vi "HFRR ADV v01.vi"() -> ()   [LabVIEW 2023] (continued)
                n759 = case shown="True" w2095 {
                  tunnel: w2094 -> [_ w2177]
                  tunnel: [FALSE ("Boolean 2") TRUE ("Boolean 2")] -> _
                  frame False {
                  }
                  frame True {
                    w2145 = ";" ("Substring")
                    # "Pid out/\nFreq response value"
                    n760 = local read "Set Strk"() -> (w2144:dbl)
                    n761 = local read "Stroke"() -> (w2134:dbl)
                    n762 = local write "act save time"(w2177) -> ()
                    n763 = Subtract(x=w2134, y=w2144) -> (x-y=w2141:dbl)
                    n764 = Multiply(x=w2141, y=0.05) -> (x*y=w2143:dbl)
                    n765 = local read "Humidity"() -> (w2152:dbl)
                    "gRh" <- w2152
                    n766 = local read "Elapsed time"() -> (w2170:dbl)
                    n767 = local read "COF 2"() -> (w2132:dbl)
                    "cof" <- w2132
                    "Coefficient of Friction" <- w2132
                    n768 = local read "AIR TEMP"() -> (w2133:dbl)
                    n769 = local read "FF 2"() -> (→"Frictional Force ( N )":dbl)
                    n770 = Add(x=w2143, y=w2144) -> (x+y=w2135:dbl)
                    "Stroke Ln" <- w2135
                    "Stroke 2" <- w2135
                    "Disp" <- w2135
                    n771 = local read "TEMP"() -> (w2129:dbl)
                    "Temp" <- w2129
                    "Electronic contact resistance ( % )" <- w2129
                    n772 = local read "ecr"() -> (w2130:dbl)
                    "ecr 2" <- w2130
                    n773 = local write "Electronic contact resistance ( % )"(w2130) -> ()
                    n774 = local read "Hz"() -> (w2137:dbl)
                    n775 = local read "PID-out"() -> (w2140:dbl)
                    n776 = Number To Fractional String(number=w2135, width (-)=i16 9 ("precision (6)"), precision (6)=i16 6) -> (F-format string=w2163:string)  [unwired: 1 in]
                    n777 = Number To Fractional String(number=w2133, width (-)=i16 9 ("precision (6)"), precision (6)=i16 3) -> (F-format string=w2162:string)  [unwired: 1 in]
                    n778 = Number To Fractional String(number=w2170, width (-)=i16 14 ("precision (6)"), precision (6)=i16 3) -> (F-format string=w2172:string)  [unwired: 1 in]
                    n779 = Number To Fractional String(number=w2132, width (-)=i16 9 ("precision (6)"), precision (6)=i16 6) -> (F-format string=w2171:string)  [unwired: 1 in]
                    n780 = Number To Fractional String(number=w2129, width (-)=i16 9 ("precision (6)"), precision (6)=i16 3) -> (F-format string=w2159:string)  [unwired: 1 in]
                    n781 = Number To Fractional String(number=w2152, width (-)=i16 9 ("precision (6)"), precision (6)=i16 3) -> (F-format string=w2156:string)  [unwired: 1 in]
                    n782 = Number To Fractional String(number=w2130, width (-)=i16 9 ("precision (6)"), precision (6)=i16 3) -> (F-format string=w2151:string)  [unwired: 1 in]
                    n783 = Number To Fractional String(number=w2140, width (-)=i16 9 ("precision (6)"), precision (6)=i16 3) -> (F-format string=w2146:string)  [unwired: 1 in]
                    n784 = Number To Fractional String(number=w2137, width (-)=i16 9 ("precision (6)"), precision (6)=i16 3) -> (F-format string=w2136:string)  [unwired: 1 in]
                    n785 = Concatenate Strings(w2172, w2145, w2171, w2145, w2163, w2145, w2162, w2145, w2159, w2145, w2156, w2145, w2151, w2145, w2146, w2145, w2136, "\r") -> (w2169:string)
                    n786 = local read "FILE"() -> (w2178:string)
                    n787 = Concatenate Strings("C:\\LAB-IQ-NXT\\Data\\" ("string"), w2178, ".dgf" ("Substring")) -> (w2180:string)
                    n788 = String To Path(string=w2180) -> (path=w2179:path)
                    n789 = call <vilib>:"Write Characters To File.vi"("append to file? (new file:F)"=TRUE, "character string"=w2169, "file path (dialog if empty)"=w2179) -> ()  [unwired: 2 in, 1 out]
                    "refresh flag" <- TRUE ("refresh flag")
                  }
                }
                n790 = local read "COUNT"() -> (w2087:i32)
                n791 = Multiply(x=w2101, y=w2087) -> (x*y=w2093:dbl)
                n792 = Add(x=w2096, y=w2093) -> (x+y=w2080:dbl)
                "Elapsed time 3" <- w2080
                n793 = local read "Test \nStatus"() -> (w2081:bool)
                n794 = local read "clk"() -> (w2088:dbl)
                n795 = Equal?(x=w2088, y=10.0) -> (x = y?=w2090:bool)
                n796 = Divide(x=w2080, y=60.0) -> (x/y=w2091:dbl)
                n797 = case shown="True" w2081 {
                  tunnel: w2091 -> [_ w2113]
                  tunnel: w2096 -> [_ w2121]
                  tunnel: [0.0 w2117] -> _
                  tunnel: w2090 -> [_ w2116]
                  tunnel: [0.0 w2115] -> _
                  tunnel: w2080 -> [_ w2115]
                  tunnel: w2094 -> [w2109 _]
                  frame False {
                    n798 = local write "acq timer"(w2109) -> ()
                  }
                  frame True {
                    n799 = local read "Set Hz"() -> (w2118:dbl)
                    n800 = local write "Elapsed time"(w2113) -> ()
                    n801 = local read "test time"() -> (w2114:dbl)
                    n802 = Multiply(x=w2121, y=w2118) -> (x*y=w2120:dbl)
                    n803 = case shown="False" w2116 {
                      tunnel: w2120 -> [w2122 _]
                      tunnel: [w2122 1.0] -> w2117
                      frame False {
                        n804 = local write "Cycles elapsed"(w2122) -> ()
                      }
                      frame True {
                      }
                    }
                    n805 = Subtract(x=w2114, y=w2113) -> (x-y=w2112:dbl)
                    "time" <- w2112
                    n806 = Greater?(x=w2113, y=w2114) -> (0:w2119:bool)
                    n807 = case shown="True" w2119 {
                      frame False {
                      }
                      frame True {
                        n808 = local read "Humidity"() -> (→"Rh After":dbl)
                        n809 = property on="STOP 2" class="Bool (strict)"("Disabled"=u8 0) -> ()  [unwired: 2 in, 2 out]
                        n810 = local write "RUN"(FALSE ("OK Button 2")) -> ()
                        n811 = local write "STOP 3"(TRUE ("STOP")) -> ()
                      }
                    }
                    n812 = local write "Time Remaining"(w2112) -> ()
                  }
                }
              }
              frame #2 {
                n813 = case shown="True" "Heater Button" {
                  tunnel: [0.0 ("output") w2204] -> w2183
                  frame False {
                    w2185 = TRUE ("tmpchk")
                    n814 = local write "tmpchk"(w2185) -> ()
                    n815 = local write "Reset 4"(w2185) -> ()
                    n816 = local read "TEMP"() -> (w2186:dbl)
                    n817 = local write "Temp ini"(w2186) -> ()
                    n818 = local write "reinit"(TRUE ("reinit")) -> ()
                  }
                  frame True {
                    # "Logic to turn off\nthe heater when \ntemp is not rising.\nTime - 60 sec\nDelta t- 5°c"
                    n819 = local read "Set Temp"() -> (w2201:dbl)
                    n820 = local read "Temp ini"() -> (w2192:dbl)
                    n821 = local read "TEMP"() -> (w2195:dbl)
                    n822 = Add(x=w2201, y=0.5) -> (x+y=w2199:dbl)
                    n823 = Less?(x=w2192, y=53.0) -> (x < y?=w2190:bool)
                    n824 = Greater Or Equal?(x=w2195, y=w2199) -> ()  [unwired: 1 out]
                    n825 = And(x="tmpchk", y=w2190) -> (x .and. y?=w2193:bool)
                    n826 = case shown="True" w2193 {
                      frame False {
                      }
                      frame True {
                        n827 = call "Elapsed Time8"("Time Target (s)"=300.0, "Reset"="Reset 4") -> ("Time has Elapsed"=w2209:bool)  [unwired: 10 in, 7 out]
                        n828 = flat-sequence {
                          tunnel: w2209 -> [_]
                          frame #0 {
                            n829 = local write "Reset 4"(FALSE ("Reset 4")) -> ()
                          }
                        }
                        n830 = case shown="True" w2209 {
                          frame False {
                          }
                          frame True {
                            n831 = local read "Temp ini"() -> (w2216:dbl)
                            n832 = local read "TEMP"() -> (w2217:dbl)
                            n833 = Add(x=w2216, y=5.0) -> (x+y=w2214:dbl)
                            n834 = Greater?(x=w2217, y=w2214) -> (0:w2215:bool)
                            n835 = case shown="False" w2215 {
                              frame False {
                                n836 = local write "Heater Button"(FALSE ("Heater Button")) -> ()
                              }
                              frame True {
                                n837 = local write "tmpchk"(FALSE ("tmpchk")) -> ()
                              }
                            }
                          }
                        }
                      }
                    }
                    n838 = call-poly <vilib>:"PID.vi"("reinitialize? (F)"="reinit", "output range"="output range", "dt (s)"=-1.0, "PID gains"="Temp PID gains", "process variable"=w2195, "setpoint"=w2201) -> ("output"=w2198:dbl)  [unwired: 4 in, 1 out]
                    n839 = Select(t=0.0, s=FALSE, f=w2198) -> (s? t:f=w2197:dbl)
                    "PID output" <- w2197
                    n840 = Subtract(x=w2201, y=w2195) -> (x-y=w2203:dbl)
                    n841 = flat-sequence {
                      tunnel: w2197 -> [w2220]
                      tunnel: [w2220] -> w2204
                      frame #0 {
                        n842 = local write "reinit"(FALSE ("reinit")) -> ()
                      }
                    }
                    n843 = Bundle(w2203, "output"=w2197, "TEMP"=w2195) -> (→"gTEMP 3":cluster{dbl, "output":dbl, "TEMP":dbl})  [unwired: 1 in]
                  }
                }
                "PID-out" <- w2183
              }
              frame #3 {
                n844 = local read "TEMP"() -> (w2222:dbl)
                n845 = Greater Or Equal?(x=w2222, y="Set Temp 2") -> (x >= y?=w2227:bool)
                n846 = case shown="True" w2227 {
                  tunnel: [FALSE TRUE] -> w2225
                  frame False {
                  }
                  frame True {
                  }
                }
                "Status 13" <- w2225
                n847 = And(x=w2225, y="trip1 8") -> (x .and. y?=w2224:bool)
                n848 = case shown="True" w2224 {
                  frame False {
                  }
                  frame True {
                    w2228 = FALSE ("OK Button 2")
                    n849 = local write "Heater Button"(w2228) -> ()
                    n850 = local write "RUN"(w2228) -> ()
                  }
                }
              }
            }
          }
        }
        n851 = stacked-sequence {
          frame #0 {
            n852 = case shown="True" "RST FF" {
              frame False {
              }
              frame True {
                w1968 = 0.0 ("X Scale.Range:Maximum")
                n853 = property on="Frictional Force ( N )" class="WFChart (strict)"("XScale.Maximum"=600.0 ("X Scale.Range:Maximum"), "XScale.Minimum"=w1968, "YScale.Maximum"=10.0 ("Y Scale.Range:Maximum"), "YScale.Minimum"=w1968) -> ()  [unwired: 2 in, 2 out]
              }
            }
          }
          frame #1 {
            n854 = case shown="True" "RST TEMP" {
              frame False {
              }
              frame True {
                n855 = property on="Temperature ( Deg C )" class="WFChart (strict)"("XScale.Minimum"=0.0 ("X Scale.Range:Minimum"), "XScale.Maximum"=600.0 ("X Scale.Range:Maximum"), "YScale.Minimum"=0.0 ("Y Scale.Range:Minimum"), "YScale.Maximum"=100.0 ("Y Scale.Range:Maximum")) -> ()  [unwired: 2 in, 2 out]
              }
            }
          }
          frame #2 {
            n856 = case shown="True" "RSTCOF" {
              frame False {
              }
              frame True {
                n857 = property on="Coefficient of Friction" class="WFChart (strict)"("XScale.Minimum"=0.0 ("X Scale.Range:Minimum"), "XScale.Maximum"=600.0 ("X Scale.Range:Maximum"), "YScale.Maximum"=1.0 ("X Scale.Range:Minimum"), "YScale.Minimum"=0.0 ("X Scale.Range:Minimum")) -> ()  [unwired: 2 in, 2 out]
              }
            }
          }
          frame #3 {
            n858 = case shown="True" "RSTCOF 2" {
              frame False {
              }
              frame True {
                (unwired) 100.0 ("Y Scale.Range:Maximum")
                (unwired) 0.0 ("Y Scale.Range:Minimum")
                (unwired) 600.0 ("X Scale.Range:Maximum")
                (unwired) 0.0 ("X Scale.Range:Minimum")
              }
            }
          }
          frame #4 {
            n859 = case shown="True" "RSTCOF 3" {
              frame False {
              }
              frame True {
                n860 = property on="Electronic contact resistance ( % )" class="WFChart (strict)"("XScale.Minimum"=0.0 ("X Scale.Range:Minimum"), "XScale.Maximum"=600.0 ("X Scale.Range:Maximum"), "YScale.Minimum"=0.0 ("Y Scale.Range:Minimum"), "YScale.Maximum"=100.0 ("Y Scale.Range:Maximum")) -> ()  [unwired: 2 in, 2 out]
              }
            }
          }
        }
        n861 = case shown="True" "Case Constant\n(See Context Help) 13" {
          frame False {
          }
          frame True {
            w1915 = TRUE ("Heater")
            n862 = local write "Rh On/Off"(w1915) -> ()
            n863 = local write "Heater Button"(w1915) -> ()
            n864 = local read "TEST STANDARD"() -> (w1918:T2)
            n865 = local read "TEST STANDARD"() -> (w1913:T2)
            n866 = Equal?(x=w1918, y=enum16{"ASTM D6079", "ISO 12156", "Custom"}."ISO 12156" ("Test Standard")) -> (x = y?=w1916:bool)
            n867 = Equal?(x=w1913, y=enum16{"ASTM D6079", "ISO 12156", "Custom"}."ASTM D6079" ("Test Standard")) -> (x = y?=w1912:bool)
            n868 = case shown="True" w1916 {
              frame False {
              }
              frame True {
                n869 = local write "airtempflg"(FALSE ("airtempflg")) -> ()
                n870 = local write "Heater"(TRUE ("Heater")) -> ()
              }
            }
            n871 = case shown="True" w1912 {
              frame False {
              }
              frame True {
                n872 = local write "airtempflg"(TRUE ("airtempflg")) -> ()
                n873 = local write "Heater"(FALSE ("Heater")) -> ()
              }
            }
          }
        }
        n874 = local read "RUN"() -> (w1859:bool)
        n875 = case shown="True" w1859 {
          tunnel: [FALSE ("TEST RUNNING") TRUE ("TEST RUNNING")] -> w1850
          frame False {
            w1989 = 0.0 ("Flag")
            n876 = local write "Flag"(w1989) -> ()
            n877 = local write "Time Remaining"(w1989) -> ()
            n878 = local write "Elapsed time"(0.0 ("elapsedtime")) -> ()
          }
          frame True {
            n879 = local write "Flag"(10.0 ("Flag")) -> ()
          }
        }
        n880 = local read "Flag"() -> (w1856:dbl)
        n881 = local read "RUN"() -> (w1853:bool)
        n882 = Equal?(x=w1856, y=10.0) -> (x = y?=w1854:bool)
        n883 = Not(x=w1853) -> (.not. x?=w1852:bool)
        n884 = And(x=w1854, y=w1852) -> (x .and. y?=w1851:bool)
        n885 = case shown="True" w1851 {
          frame False {
          }
          frame True {
            w1966 = FALSE ("Heater Button")
            n886 = local write "Heater Button"(w1966) -> ()
            n887 = local write "Rh On/Off"(w1966) -> ()
          }
        }
        n888 = local write "Save"(w1850) -> ()
        n889 = local write "Test \nStatus"(w1850) -> ()
        n890 = local write "st enable"(w1850) -> ()
        n891 = local write "PWR"(w1850) -> ()
        n892 = local read "Set Temp"() -> (w1812:dbl)
        n893 = local read "SetTemp"() -> (w1814:dbl)
        n894 = local read "Set Rh"() -> (w1813:dbl)
        n895 = local read "Amb temp"() -> (w1811:dbl)
        n896 = local read "Humidity"() -> (w1810:dbl)
        n897 = local read "TEMP"() -> (w1809:dbl)
        n898 = Add(x=w1814, y=w1839) -> (x+y=w1840:dbl)
        n899 = Subtract(x=w1814, y=w1839) -> (x-y=w1841:dbl)
        n900 = Add(x=w1813, y=w1838) -> (x+y=w1837:dbl)
        n901 = Subtract(x=w1813, y=w1838) -> (x-y=w1836:dbl)
        n902 = Add(x=w1812, y=w1833) -> (x+y=w1834:dbl)
        n903 = Subtract(x=w1812, y=w1833) -> (x-y=w1835:dbl)
        n904 = In Range and Coerce(upper limit=w1840, x=w1811, lower limit=w1841) -> (In Range?=w1830:bool)  [unwired: 1 out]
        n905 = In Range and Coerce(upper limit=w1837, x=w1810, lower limit=w1836) -> (In Range?=w1828:bool)  [unwired: 1 out]
        n906 = In Range and Coerce(upper limit=w1834, x=w1809, lower limit=w1835) -> (In Range?=w1826:bool)  [unwired: 1 out]
        n907 = case shown="True" w1830 {
          tunnel: [FALSE ("RUN") TRUE ("RUN")] -> w1829
          tunnel: [_ 1] -> w1822
          frame False {
          }
          frame True {
          }
        }
        n908 = case shown="True" w1828 {
          tunnel: [FALSE ("RUN") TRUE ("RUN")] -> w1827
          tunnel: [_ 2] -> w1821
          frame False {
          }
          frame True {
          }
        }
        n909 = case shown="True" w1826 {
          tunnel: [FALSE ("RUN") TRUE ("RUN")] -> w1825
          tunnel: [_ 3] -> w1820
          frame False {
          }
          frame True {
          }
        }
        n910 = local read "airtempflg"() -> (w1831:bool)
        n911 = Or(x=w1831, y=w1829) -> (x .or. y?=w1832:bool)
        n912 = Build Array(w1822, w1821, w1820) -> (w1818:i32[])
        n913 = Compound Arithmetic op=AND(w1832, w1827, w1825) -> ()  [unwired: 1 out]
        n914 = case shown="True" "Case Constant\n(See Context Help) 14" {
          frame False {
          }
          frame True {
            w1909 = FALSE ("autostrtflg")
            n915 = local write "autostrtflg"(w1909) -> ()
            n916 = local write "autostart"(w1909) -> ()
            n917 = local write "RUN"(TRUE ("RUN")) -> ()
            n918 = local write "String 14"(" Running....." ("String 14")) -> ()
          }
        }
        n919 = Insert Into Array(array=string[] ["Air Temperature has reached set value,", "Humidity has reached set value,", "Sample Temperaturehas reached set value,", ""], index=0, new element="") -> (w1817:string[])
        n920 = for {
          tunnel: w1818 -> [w1899] mode=indexing
          tunnel: w1817 -> [w1898]
          shift-right: [w1895] -> w1816
          shift-left: "" -> [w1897]
          n921 = Index Array(array=w1898, index=w1899) -> (element=w1896:string)
          n922 = Concatenate Strings(w1896, w1897) -> (w1895:string)
        }
        n923 = local write "autostart 2"(w1816) -> ()
      }
      frame 1 {
        # "Elapsed time\ncof\nstroke\nAir temp\nTemp\nHumidity"
        n924 = case shown="True" "OPEN 4" {
          frame False {
          }
          frame True {
            (unwired) 0  # existing file
            w2419 = "Choose a datalog file to open"  # prompt
            n925 = local write "OPEN 4"(FALSE ("OPEN 1")) -> ()
            n926 = String To Path(string="C:\\LAB-IQ-NXT\\Data\\") -> (path=w2404:path)
            n927 = File Dialog(6:"*.dgf" ("pattern"), 7:w2419, 11:w2404) -> (0:w2402:errorcluster, 3:w2410:path)  [unwired: 4 in, 2 out]
            n928 = Unbundle(w2402) -> ()  [unwired: 3 out]
            n929 = Path To String(path=w2410) -> (string=w2405:string)
            "string1 4" <- w2405
            n930 = Match Pattern(string=w2405, regular expression=".dgf" ("substring (\"\")")) -> (before substring=w2415:string)  [unwired: 1 in, 3 out]
            n931 = Concatenate Strings(w2415, ".duf" ("Substring")) -> (w2412:string)
            n932 = String To Path(string=w2412) -> (path=w2416:path)
            n933 = call <vilib>:"Read Characters From File.vi"("file path (dialog if empty)"=w2416, "start of read offset (chars.:0)"=60 ("start of read offset (chars.: 0)")) -> ("character string"=→"String Control 8":string)  [unwired: 4 in, 3 out]
            n934 = Strip Path(path=w2410) -> (name=w2408:string)  [unwired: 1 out]
            n935 = Match Pattern(string=w2408, regular expression=".dgf") -> (before substring=→"String Control 7":string)  [unwired: 1 in, 3 out]
          }
        }
        n936 = case shown="True" "OPEN 3" {
          frame False {
          }
          frame True {
            (unwired) 0  # existing file
            w2401 = "Choose a datalog file to open"  # prompt
            n937 = local write "OPEN 3"(FALSE ("OPEN 1")) -> ()
            n938 = String To Path(string="C:\\LAB-IQ-NXT\\Data\\") -> (path=w2386:path)
            n939 = File Dialog(6:"*.dgf" ("pattern"), 7:w2401, 11:w2386) -> (0:w2384:errorcluster, 3:w2392:path)  [unwired: 4 in, 2 out]
            n940 = Unbundle(w2384) -> ()  [unwired: 3 out]
            n941 = Path To String(path=w2392) -> (string=w2387:string)
            "string1 3" <- w2387
            n942 = Match Pattern(string=w2387, regular expression=".dgf" ("substring (\"\")")) -> (before substring=w2397:string)  [unwired: 1 in, 3 out]
            n943 = Concatenate Strings(w2397, ".duf" ("Substring")) -> (w2394:string)
            n944 = String To Path(string=w2394) -> (path=w2398:path)
            n945 = call <vilib>:"Read Characters From File.vi"("file path (dialog if empty)"=w2398, "start of read offset (chars.:0)"=60 ("start of read offset (chars.: 0)")) -> ("character string"=→"String Control 6":string)  [unwired: 4 in, 3 out]
            n946 = Strip Path(path=w2392) -> (name=w2390:string)  [unwired: 1 out]
            n947 = Match Pattern(string=w2390, regular expression=".dgf") -> (before substring=→"String Control 5":string)  [unwired: 1 in, 3 out]
          }
        }
        n948 = case shown="True" "OPEN 2" {
          frame False {
          }
          frame True {
            (unwired) 0  # existing file
            w2383 = "Choose a datalog file to open"  # prompt
            n949 = local write "OPEN 2"(FALSE ("OPEN 1")) -> ()
            n950 = String To Path(string="C:\\LAB-IQ-NXT\\Data\\") -> (path=w2368:path)
            n951 = File Dialog(6:"*.dgf" ("pattern"), 7:w2383, 11:w2368) -> (0:w2366:errorcluster, 3:w2374:path)  [unwired: 4 in, 2 out]
            n952 = Unbundle(w2366) -> ()  [unwired: 3 out]
            n953 = Path To String(path=w2374) -> (string=w2369:string)
            "string1 2" <- w2369
            n954 = Match Pattern(string=w2369, regular expression=".dgf" ("substring (\"\")")) -> (before substring=w2380:string)  [unwired: 1 in, 3 out]
            n955 = Concatenate Strings(w2380, ".duf" ("Substring")) -> (w2377:string)
            n956 = String To Path(string=w2377) -> (path=w2375:path)
            n957 = call <vilib>:"Read Characters From File.vi"("file path (dialog if empty)"=w2375, "start of read offset (chars.:0)"=60 ("start of read offset (chars.: 0)")) -> ("character string"=→"String Control 4":string)  [unwired: 4 in, 3 out]
            n958 = Strip Path(path=w2374) -> (name=w2372:string)  [unwired: 1 out]
            n959 = Match Pattern(string=w2372, regular expression=".dgf") -> (before substring=→"String Control 3":string)  [unwired: 1 in, 3 out]
          }
        }
        n960 = case shown="True" "OPEN 1" {
          frame False {
          }
          frame True {
            (unwired) 0  # existing file
            w2365 = "Choose a datalog file to open"  # prompt
            n961 = local write "OPEN 1"(FALSE ("OPEN 1")) -> ()
            n962 = String To Path(string="C:\\LAB-IQ-NXT\\Data\\") -> (path=w2350:path)
            n963 = File Dialog(6:"*.dgf" ("pattern"), 7:w2365, 11:w2350) -> (0:w2348:errorcluster, 3:w2356:path)  [unwired: 4 in, 2 out]
            n964 = Unbundle(w2348) -> ()  [unwired: 3 out]
            n965 = Path To String(path=w2356) -> (string=w2351:string)
            "string1" <- w2351
            n966 = Match Pattern(string=w2351, regular expression=".dgf" ("substring (\"\")")) -> (before substring=w2361:string)  [unwired: 1 in, 3 out]
            n967 = Concatenate Strings(w2361, ".duf" ("Substring")) -> (w2357:string)
            n968 = String To Path(string=w2357) -> (path=w2362:path)
            n969 = call <vilib>:"Read Characters From File.vi"("file path (dialog if empty)"=w2362, "start of read offset (chars.:0)"=60 ("start of read offset (chars.: 0)")) -> ("character string"=→"String Control 2":string)  [unwired: 4 in, 3 out]
            n970 = Strip Path(path=w2356) -> (name=w2355:string)  [unwired: 1 out]
            n971 = Match Pattern(string=w2355, regular expression=".dgf") -> (before substring=→"String Control":string)  [unwired: 1 in, 3 out]
          }
        }
        n972 = case shown="True" "RSTV1 4" {
          frame False {
          }
          frame True {
            n973 = property on="XY Graph 14" class="XYGraph (strict)"("Y Scale.Display Format:Precision"=u8 2 ("Y Scale.Format & Precision:Precision")) -> ()  [unwired: 2 in, 2 out]
            n974 = property on="XY Graph 14" class="XYGraph (strict)"("X Scale.Range:Minimum"=0.0 ("Y Scale.Range:Maximum"), "X Scale.Range:Maximum"=75.0 ("X Scale.Range:Minimum"), "Y Scale.Range:Minimum"=0.98, "Y Scale.Range:Maximum"=1.02) -> ()  [unwired: 2 in, 2 out]
          }
        }
        n975 = case shown="True" "rstv2" {
          frame False {
          }
          frame True {
            n976 = property on="XY Graph 9" class="XYGraph (strict)"("X Scale.Range:Minimum"=0.0 ("Y Scale.Range:Maximum"), "X Scale.Range:Maximum"=75.0, "Y Scale.Range:Minimum"=0.0, "Y Scale.Range:Maximum"=1.0 ("X Scale.Range:Minimum")) -> ()  [unwired: 2 in, 2 out]
            n977 = property on="XY Graph 9" class="XYGraph (strict)"("Y Scale.Display Format:Precision"=u8 3 ("Y Scale.Format & Precision:Precision")) -> ()  [unwired: 2 in, 2 out]
          }
        }
        n978 = case shown="True" "RSTV1 3" {
          frame False {
          }
          frame True {
            n979 = property on="XY Graph 10" class="XYGraph (strict)"("X Scale.Range:Minimum"=0.0 ("Y Scale.Range:Minimum"), "X Scale.Range:Maximum"=75.0 ("Y Scale.Range:Maximum"), "Y Scale.Range:Minimum"=20.0 ("X Scale.Range:Minimum"), "Y Scale.Range:Maximum"=26.0 ("X Scale.Range:Maximum")) -> ()  [unwired: 2 in, 2 out]
            n980 = property on="XY Graph 10" class="XYGraph (strict)"("Y Scale.Display Format:Precision"=u8 2 ("Y Scale.Format & Precision:Precision")) -> ()  [unwired: 2 in, 2 out]
          }
        }
        n981 = case shown="True" "RST CP" {
          frame False {
          }
          frame True {
            n982 = property on="XY Graph 12" class="XYGraph (strict)"("X Scale.Range:Minimum"=0.0, "X Scale.Range:Maximum"=75.0, "Y Scale.Range:Minimum"=58.0, "Y Scale.Range:Maximum"=62.0) -> ()  [unwired: 2 in, 2 out]
            n983 = property on="XY Graph 12" class="XYGraph (strict)"("Y Scale.Display Format:Precision"=u8 2 ("Y Scale.Format & Precision:Precision")) -> ()  [unwired: 2 in, 2 out]
          }
        }
        n984 = case shown="True" "RST CP 2" {
          frame False {
          }
          frame True {
            n985 = property on="XY Graph 13" class="XYGraph (strict)"("X Scale.Range:Minimum"=0.0, "X Scale.Range:Maximum"=75.0, "Y Scale.Range:Minimum"=0.0, "Y Scale.Range:Maximum"=100.0) -> ()  [unwired: 2 in, 2 out]
            n986 = property on="XY Graph 13" class="XYGraph (strict)"("Y Scale.Display Format:Precision"=u8 0 ("Y Scale.Format & Precision:Precision")) -> ()  [unwired: 2 in, 2 out]
          }
        }
        n987 = case shown="True" "RSTV1 2" {
          frame False {
          }
          frame True {
            n988 = property on="XY Graph 11" class="XYGraph (strict)"("X Scale.Range:Minimum"=0.0, "X Scale.Range:Maximum"=75.0, "Y Scale.Range:Minimum"=48.0, "Y Scale.Range:Maximum"=58.0) -> ()  [unwired: 2 in, 2 out]
            n989 = property on="XY Graph 11" class="XYGraph (strict)"("Y Scale.Display Format:Precision"=u8 0 ("Y Scale.Format & Precision:Precision")) -> ()  [unwired: 2 in, 2 out]
          }
        }
        n990 = case shown="True" "RST CP 3" {
          frame False {
          }
          frame True {
            n991 = property on="XY Graph 15" class="XYGraph (strict)"("X Scale.Range:Minimum"=18.0, "X Scale.Range:Maximum"=28.0 ("X Scale.Range:Minimum"), "Y Scale.Range:Minimum"=30.0 ("X Scale.Range:Minimum"), "Y Scale.Range:Maximum"=70.0 ("X Scale.Range:Minimum")) -> ()  [unwired: 2 in, 2 out]
          }
        }
      }
      frame 2 {
        # "Elapsed time\ncof\nstroke\nmean pos\nTemp\nHumidity"
        n992 = case shown="True" "Export" {
          frame False {
          }
          frame True {
            w2550 = "                                      " ("string")
            w2552 = "\r"
            (unwired) i16 6 ("width (-)")
            w2629 = "\r"
            w2561 = "\r"
            n993 = local read "Sample ID"() -> (w2636:string)
            n994 = local read "Temperature after test 2"() -> (w2623:dbl)
            n995 = local read "Test Date"() -> (w2635:string)
            n996 = local read "String 45"() -> (w2549:string)
            n997 = local read "String 32"() -> (w2633:string)
            n998 = local read "String 31"() -> (w2634:string)
            n999 = local read "String 38"() -> (w2571:string)
            n1000 = local read "Humidity after test 2"() -> (w2619:dbl)
            n1001 = local read "s.NO"() -> (w2551:string)
            n1002 = local read "String 36"() -> (w2574:string)
            n1003 = local read "Temperature before test 2"() -> (w2618:dbl)
            n1004 = local read "String 37"() -> (w2577:string)
            n1005 = local read "AVP 2"() -> (w2616:dbl)
            n1006 = local read "HCF 2"() -> (w2627:dbl)
            n1007 = local read "MWSD 2"() -> (w2615:dbl)
            n1008 = local read "String 35"() -> (w2581:string)
            n1009 = local write "Export"(FALSE ("Export")) -> ()
            n1010 = local read "Humidity before test 2"() -> (w2604:dbl)
            n1011 = Concatenate Strings("7," ("string"), w2571) -> (w2572:string)
            n1012 = Concatenate Strings("6," ("string"), w2574) -> (w2575:string)
            n1013 = local read "S 39"() -> (w2582:string)
            n1014 = Concatenate Strings("5," ("string"), w2577) -> (w2578:string)
            n1015 = local read "String 34"() -> (w2586:string)
            n1016 = Concatenate Strings("4," ("string"), w2581) -> (w2580:string)
            n1017 = Concatenate Strings("3," ("string"), w2582) -> (w2584:string)
            n1018 = local read "S 38"() -> (w2589:string)
            n1019 = Number To Fractional String(number=w2627, width (-)=i16 6, precision (6)=i16 2) -> (F-format string=w2628:string)  [unwired: 1 in]
            n1020 = Number To Fractional String(number=w2615, width (-)=i16 6, precision (6)=i16 2) -> (F-format string=w2613:string)  [unwired: 1 in]
            n1021 = Number To Fractional String(number=w2616, width (-)=i16 6, precision (6)=i16 2) -> (F-format string=w2614:string)  [unwired: 1 in]
            n1022 = Number To Fractional String(number=w2623, width (-)=i16 6, precision (6)=i16 2) -> (F-format string=w2622:string)  [unwired: 1 in]
            n1023 = Number To Fractional String(number=w2619, width (-)=i16 6, precision (6)=i16 2) -> (F-format string=w2617:string)  [unwired: 1 in]
            n1024 = Number To Fractional String(number=w2618, width (-)=i16 6, precision (6)=i16 2) -> (F-format string=w2624:string)  [unwired: 1 in]
            n1025 = Number To Fractional String(number=w2604, width (-)=i16 6, precision (6)=i16 2) -> (F-format string=w2603:string)  [unwired: 1 in]
            n1026 = local read "String 39"() -> (w2568:string)
            n1027 = Concatenate Strings("2," ("string"), w2586) -> (w2585:string)
            n1028 = local read "WS1.4 2"() -> (w2631:dbl)
            n1029 = Concatenate Strings(w2561, "," ("string"), w2549, w2551, w2550, w2633, w2636, w2550, w2634, w2635, w2561) -> (w2559:string)
            n1030 = Concatenate Strings("1," ("string"), w2589) -> (w2588:string)
            n1031 = Concatenate Strings("8," ("string"), w2568) -> (w2569:string)
            n1032 = Number To Fractional String(number=w2631, precision (6)=i16 2) -> (F-format string=w2632:string)  [unwired: 2 in]
            n1033 = Concatenate Strings(w2629, w2588, w2603, w2629, w2585, w2624, w2629, w2584, w2617, w2629, w2580, w2622, w2629, w2578, w2613, w2629, w2575, w2614, w2629, w2572, w2628, w2629, w2569, w2632) -> (w2591:string)
            n1034 = Concatenate Strings("S.No," ("string"), "                                       Parameters" ("string")) -> (w2562:string)
            n1035 = local read "TITTLE"() -> (w2557:string)
            n1036 = local read "String 33"() -> (w2566:string)
            n1037 = local read "Tested by"() -> (w2565:string)
            n1038 = Concatenate Strings("=" ("string"), w2557) -> (w2556:string)
            n1039 = local read "String 29"() -> (w2598:string)
            n1040 = Concatenate Strings("," ("string"), "                                                                             " ("string")) -> (w2554:string)
            n1041 = Concatenate Strings(w2556, w2552, w2559, w2552, w2562, w2591, w2552, w2554, w2566, w2565) -> (→"export":string)
            n1042 = Match Pattern(string=w2598, regular expression=".dwm") -> (before substring=w2594:string)  [unwired: 1 in, 3 out]
            "before substring" <- w2594
            n1043 = case shown="\"xlx\"" "Select File Type" {
              tunnel: w2594 -> [w2639 w2641 w2643]
              tunnel: [w2637 w2642 w2644] -> w2593
              frame "xlx" {
                n1044 = Concatenate Strings(w2639, ".xls" ("string")) -> (w2637:string)
              }
              frame "csv" {
                n1045 = Concatenate Strings(w2641, ".csv" ("string")) -> (w2642:string)
              }
              frame "txt" {
                n1046 = Concatenate Strings(w2643, ".txt" ("string")) -> (w2644:string)
              }
            }
            n1047 = String To Path(string=w2593) -> (path=w2600:path)
            n1048 = local read "export"() -> (w2595:string)
            n1049 = call <vilib>:"Write Characters To File.vi"("append to file? (new file:F)"=FALSE, "character string"=w2595, "file path (dialog if empty)"=w2600) -> ()  [unwired: 2 in, 1 out]
          }
        }
        n1050 = case shown="True" "OK Button 16" {
          frame False {
          }
          frame True {
            n1051 = stacked-sequence {
              frame #0 {
                n1052 = local read "Numeric 16"() -> (w2759:i32)
                n1053 = local write "Numeric 10"(w2759) -> ()
              }
              frame #1 {
                n1054 = local read "String 29"() -> (w2763:string)
                n1055 = String To Path(string=w2763) -> (path=w2762:path)
                n1056 = local read "S.NO"() -> (→"s.NO":string)
                n1057 = Open/Create/Replace File "Open File"(file path (use dialog)=w2762) -> (refnum out=w2764:refnum<file>)  [unwired: 5 in, 2 out]
                n1058 = for {
                  N: 16 -> [_]
                  tunnel: w2764 -> [w2771]
                  i -> [w2767]
                  (unwired) TRUE ("line mode (F)")
                  n1059 = Read from Text File "Read File"(file (use dialog)=w2771) -> (text=w2765:string)  [unwired: 3 in, 3 out]
                  n1060 = Match Pattern(string=w2765, regular expression="(") -> (after substring=w2770:string)  [unwired: 1 in, 3 out]
                  n1061 = Match Pattern(string=w2770, regular expression=")") -> (before substring=w2766:string)  [unwired: 1 in, 3 out]
                  n1062 = case shown="1" w2767 {
                    tunnel: w2766 -> [w2772 w2773 _ _ w2774 w2775 w2776 w2778 w2780 w2782 w2784 w2786 w2788 w2790 _]
                    tunnel: w2765 -> [_ _ _ _ _ _ _ _ _ _ _ _ _ _ _]
                    frame 0 {
                      "TITTLE" <- w2772
                    }
                    frame 1 {
                      "Sample ID" <- w2773
                    }
                    frame 2 {
                    }
                    frame 3 {
                    }
                    frame 4 {
                      "Test Date" <- w2774
                    }
                    frame 5 {
                      "Tested by" <- w2775
                    }
                    frame 6 {
                      n1063 = Fract/Exp String To Number(string=w2776) -> (number=→"Humidity before test 2":dbl)  [unwired: 3 in, 1 out]
                    }
                    frame 7 {
                      n1064 = Fract/Exp String To Number(string=w2778) -> (number=→"Temperature before test 2":dbl)  [unwired: 3 in, 1 out]
                    }
                    frame 8 {
                      n1065 = Fract/Exp String To Number(string=w2780) -> (number=→"Humidity after test 2":dbl)  [unwired: 3 in, 1 out]
                    }
                    frame 9 {
                      n1066 = Fract/Exp String To Number(string=w2782) -> (number=→"Temperature after test 2":dbl)  [unwired: 3 in, 1 out]
                    }
                    frame 10 {
                      n1067 = Fract/Exp String To Number(string=w2784) -> (number=→"MWSD 2":dbl)  [unwired: 3 in, 1 out]
                    }
                    frame 11 {
                      n1068 = Fract/Exp String To Number(string=w2786) -> (number=→"AVP 2":dbl)  [unwired: 3 in, 1 out]
                    }
                    frame 12 {
                      n1069 = Fract/Exp String To Number(string=w2788) -> (number=→"HCF 2":dbl)  [unwired: 3 in, 1 out]
                    }
                    frame 13 {
                      n1070 = Fract/Exp String To Number(string=w2790) -> (number=→"WS1.4 2":dbl)  [unwired: 3 in, 1 out]
                    }
                    frame 14, Default {
                    }
                  }
                }
              }
              frame #2 {
              }
            }
            n1071 = local write "OK Button 16"(FALSE ("OK Button 13")) -> ()
          }
        }
        n1072 = call <vilib>:"Query Available Printers.vi"() -> ("system configured printers"=w2434:string[])  [unwired: 9 in, 2 out]
        "System Configured Printers 2" <- w2434
        n1073 = Index Array(array=w2434, index="Select Printer 3") -> (element=w2436:string)
        "Selected Printer" <- w2436
        n1074 = case shown="True" "Print 2" {
          frame False {
          }
          frame True {
            n1075 = flat-sequence {
              frame #0 {
                n1076 = local read "Ref A Test Date :"() -> (→"TITTLE 4":string)
                n1077 = local read "Sample ID"() -> (→"Sample ID  2":string)
                n1078 = local read "s.NO"() -> (→"s.NO 2":string)
                n1079 = local read "Test Date"() -> (→"Test Date 2":string)
                n1080 = local read "Tested by"() -> (→"Tested by 2":string)
                n1081 = local read "Temperature before test 3"() -> (w2454:dbl)
                n1082 = local read "Temperature before test 3"() -> (→"Temperature after test 5":dbl)
                n1083 = local read "Temperature after test 3"() -> (→"Temperature after test 4":dbl)
                n1084 = local read "Sample ID  3"() -> (→"Sample ID  6":string)
                n1085 = local read "Sample ID  4"() -> (→"Sample ID  7":string)
                n1086 = local read "Humidity before test 3"() -> (→"Humidity before test 4":dbl)
                n1087 = local read "Humidity after test 3"() -> (→"Humidity after test 4":dbl)
                n1088 = local write "Temperature before test 3"(w2454) -> ()
                n1089 = String To Path(string="C:\\LAB-IQ-NXT\\im\\Temp_resized.jpg") -> (path=w2446:path)
                "path 2" <- w2446
                n1090 = local read "image data"() -> (w2445:T5)
                n1091 = Wait (ms)(milliseconds to wait=u32 20) -> ()  [unwired: 1 out]
                n1092 = call <vilib>:"Write JPEG File.vi"("image data"=w2445, "path to JPEG file"=w2446) -> ()  [unwired: 8 in, 2 out]
                "Ref A Test Date :" <- "Ref A Test Date :"
                "Ref B Test Date :" <- "Ref B Test Date :"
                "Ref B Scar Value :" <- "Ref B Scar Value :"
                "Ref A Scar Value :" <- "Ref A Scar Value :"
              }
              frame #1 {
                (unwired) HTML_Report_Image_Alignment."MIDDLE" ("alignment (default)")
                w2482 = u16 0 items=["portrait", "landscape"] ("orientation (portrait)")
                (unwired) HTML_Report_Image_Alignment."ABSMIDDLE" ("alignment (default)")
                (unwired) "TESTED BY : "
                (unwired) "TESTED DATE :"
                (unwired) "SAMPLE ID : "
                (unwired) "SAMPLE DESIGN : "
                w2515 = "\r"
                # "add image"
                n1093 = call <vilib>:"New Report.vi"("report type"=enum16{"Standard Report", "HTML"}."HTML") -> ("report out"=w2486:refnum<class "NI_report.lvclass">, "error out"=w2484:errorcluster)  [unwired: 13 in]
                n1094 = Wait (ms)(milliseconds to wait=u32 20) -> ()  [unwired: 1 out]
                n1095 = call-dynamic "Set Report Orientation.vi"("report in"=w2486, "orientation (portrait)"=w2482, "error in (no error)"=w2484) -> ("report out"=w2485:refnum<class "NI_report.lvclass">, "error out"=w2483:errorcluster)  [unwired: 11 in]
                n1096 = for {
                  N: 5 -> [_]
                  tunnel: w2485 -> [w2536]
                  tunnel: [w2535] -> w2464
                  tunnel: w2483 -> [w2534]
                  tunnel: [w2533] -> w2463
                  n1097 = call-dynamic "Set Report Tab Width.vi"("report in"=w2536, "error in (no error)"=w2534) -> ("report out"=w2535:refnum<class "NI_report.lvclass">, "error out"=w2533:errorcluster)  [unwired: 12 in]
                }
                n1098 = local read "Sample ID  2"() -> (w2508:string)
                n1099 = local read "s.NO 2"() -> (w2507:string)
                n1100 = local read "Test Date 2"() -> (w2509:string)
                n1101 = local read "Tested by 2"() -> (w2510:string)
                n1102 = local read "String 46"() -> (w2506:string)
                n1103 = local read "String 48"() -> (w2512:string)
                n1104 = local read "String 47"() -> (w2511:string)
                n1105 = local read "String 49"() -> (w2513:string)
                n1106 = local read "TITTLE"() -> (w2481:string)
                n1107 = call-dynamic "Set Report Header Text.vi"("report in"=w2464, "center header text"=w2481, "error in (no error)"=w2463) -> ("report out"=w2502:refnum<class "NI_report.lvclass">, "error out"=w2501:errorcluster)  [unwired: 11 in]
                n1108 = for {
                  N: 1 -> [_]
                  tunnel: [w2540] -> w2488
                  tunnel: [w2539] -> w2487
                  tunnel: w2502 -> [w2538]
                  tunnel: w2501 -> [w2537]
                  n1109 = call-dynamic "New Report Line.vi"("report in"=w2538, "error in (no error)"=w2537) -> ("report out"=w2540:refnum<class "NI_report.lvclass">, "error out"=w2539:errorcluster)  [unwired: 12 in]
                }
                n1110 = Concatenate Strings(w2515, w2506, w2507, w2515, w2512, w2508, w2515, w2511, w2509, w2515, w2513, w2510, w2515) -> (→"test by 2":string)
                n1111 = for {
                  N: 2 -> [_]
                  tunnel: [w2532] -> w2494
                  tunnel: [w2531] -> w2493
                  tunnel: w2488 -> [w2530]
                  tunnel: w2487 -> [w2529]
                  n1112 = call-dynamic "New Report Line.vi"("report in"=w2530, "error in (no error)"=w2529) -> ("report out"=w2532:refnum<class "NI_report.lvclass">, "error out"=w2531:errorcluster)  [unwired: 12 in]
                }
                n1113 = for {
                  N: 25 -> [_]
                  tunnel: w2494 -> [w2528]
                  tunnel: w2493 -> [w2526]
                  tunnel: [w2527] -> w2497
                  tunnel: [w2525] -> w2496
                  n1114 = call-dynamic "Set Report Tab Width.vi"("report in"=w2528, "error in (no error)"=w2526) -> ("report out"=w2527:refnum<class "NI_report.lvclass">, "error out"=w2525:errorcluster)  [unwired: 12 in]
                }
                n1115 = control-ref of="Tab Control 9"() -> (w2492:refnum<vi>)
                n1116 = local read "Wear Scar X"() -> (w2480:dbl)
                "Length ( microns ) 2" <- w2480
                n1117 = local read "Wear Scar Y"() -> (w2479:dbl)
                "Wear Scar Y ( microns ) :" <- w2479
                n1118 = call-dynamic "Append Control Image to Report.vi"("report in"=w2497, "alignment (default)"=HTML_Report_Image_Alignment."ABSMIDDLE", "ctrl reference"=w2492, "error in (no error)"=w2496) -> ("report out"=w2491:refnum<class "NI_report.lvclass">, "error out"=w2490:errorcluster)  [unwired: 8 in, 2 out]
                n1119 = for {
                  N: 3 -> [_]
                  tunnel: [w2524] -> w2475
                  tunnel: [w2523] -> w2474
                  tunnel: w2491 -> [w2522]
                  tunnel: w2490 -> [w2521]
                  n1120 = call-dynamic "New Report Line.vi"("report in"=w2522, "error in (no error)"=w2521) -> ("report out"=w2524:refnum<class "NI_report.lvclass">, "error out"=w2523:errorcluster)  [unwired: 12 in]
                }
                n1121 = Add(x=w2480, y=w2479) -> (x+y=w2478:dbl)
                n1122 = Divide(x=w2478, y=2.0) -> (x/y=→"Mean Wear ( microns) :":dbl)
                n1123 = local read "String 10"() -> (w2466:string)
                n1124 = for {
                  N: 100 -> [_]
                  tunnel: w2475 -> [w2520]
                  tunnel: w2474 -> [w2518]
                  tunnel: [w2519] -> w2471
                  tunnel: [w2517] -> w2469
                  n1125 = call-dynamic "Set Report Tab Width.vi"("report in"=w2520, "error in (no error)"=w2518) -> ("report out"=w2519:refnum<class "NI_report.lvclass">, "error out"=w2517:errorcluster)  [unwired: 12 in]
                }
                n1126 = Concatenate Strings("C:\\LAB-IQ-NXT\\Data\\" ("string"), w2466, ".jpg" ("string")) -> ()  [unwired: 1 out]
                n1127 = String To Path(string="C:\\LAB-IQ-NXT\\im\\Temp_resized.jpg") -> (path=w2461:path)
                n1128 = call-poly <vilib>:"Append Image to Report.vi"("report in"=w2471, "path or URL of image"=w2461, "error in (no error)"=w2469) -> ("report out"=w2470:refnum<class "NI_report.lvclass">, "error out"=w2468:errorcluster)  [unwired: 9 in, 2 out]
                n1129 = call-poly <vilib>:"Open HTML Report in Browser.vi"("report in"=w2470, "error in (no error)"=w2468) -> ("report out"=w2505:refnum<class "NI_report.lvclass">, "error out"=w2504:errorcluster)  [unwired: 11 in, 1 out]
                n1130 = call-dynamic "Dispose Report.vi"("report in"=w2505, "error in (no error)"=w2504) -> ()  [unwired: 13 in, 1 out]
              }
              frame #2 {
              }
              frame #3 {
                n1131 = case shown="True" "Case Constant\n(See Context Help) 16" {
                  frame False {
                  }
                  frame True {
                    n1132 = local read "String 10"() -> (w2546:string)
                    n1133 = Concatenate Strings("C:\\LAB-IQ-NXT\\Data\\" ("string"), w2546, ".jpg" ("string")) -> (w2544:string)
                    n1134 = String To Path(string=w2544) -> (path=w2543:path)
                    n1135 = Delete(path (use dialog)=w2543) -> ()  [unwired: 4 in, 3 out]
                  }
                }
                n1136 = local write "Print 2"(FALSE ("Print")) -> ()
              }
            }
          }
        }
        n1137 = local read "OK Button 16"() -> (w2430:bool)
        n1138 = case shown="True" "Print" {
          tunnel: w2436 -> [_ w2728]
          frame False {
          }
          frame True {
            (unwired) i16 6 ("width (-)")
            (unwired) "TESTED BY : "
            (unwired) "TESTED DATE :"
            (unwired) "SAMPLE ID : "
            (unwired) "SAMPLE DESIGN : "
            w2686 = "\r"
            w2703 = "\r"
            # "add image"
            n1139 = local read "String 45"() -> (w2646:string)
            n1140 = local read "Sample ID"() -> (w2676:string)
            n1141 = local read "Tested by"() -> (w2679:string)
            n1142 = local read "Test Date"() -> (w2677:string)
            n1143 = local read "String 32"() -> (w2681:string)
            n1144 = local read "String 31"() -> (w2680:string)
            n1145 = local read "String 33"() -> (w2682:string)
            n1146 = local read "s.NO"() -> (w2647:string)
            n1147 = call <vilib>:"New Report.vi"("report type"=enum16{"Standard Report", "HTML"}."Standard Report") -> ("report out"=w2726:refnum<class "NI_report.lvclass">, "error out"=w2725:errorcluster)  [unwired: 13 in]
            n1148 = local read "TITTLE"() -> (w2678:string)
            n1149 = call-dynamic "Set Report Header Text.vi"("report in"=w2726, "center header text"=w2678, "error in (no error)"=w2725) -> ("report out"=w2697:refnum<class "NI_report.lvclass">, "error out"=w2698:errorcluster)  [unwired: 11 in]
            n1150 = Concatenate Strings(w2703, w2646, w2647, w2703, w2681, w2676, w2703, w2680, w2677, w2703, w2682, w2679, w2703) -> (w2696:string)
            "test by" <- w2696
            n1151 = local read "Temperature after test 2"() -> (w2692:dbl)
            n1152 = local read "String 38"() -> (w2652:string)
            n1153 = local read "Humidity after test 2"() -> (w2701:dbl)
            n1154 = local read "String 36"() -> (w2656:string)
            n1155 = local read "Temperature before test 2"() -> (w2702:dbl)
            n1156 = local read "String 37"() -> (w2659:string)
            n1157 = local read "AVP 2"() -> (w2705:dbl)
            n1158 = local read "HCF 2"() -> (w2688:dbl)
            n1159 = local read "MWSD 2"() -> (w2706:dbl)
            n1160 = local read "String 35"() -> (w2661:string)
            n1161 = call-poly <vilib>:"Append Report Text.vi"("report in"=w2697, "text"=w2696, "error in (no error)"=w2698) -> ("report out"=w2700:refnum<class "NI_report.lvclass">, "error out"=w2699:errorcluster)  [unwired: 9 in, 2 out]
            n1162 = local read "Humidity before test 2"() -> (w2717:dbl)
            n1163 = Concatenate Strings("7)" ("string"), w2652) -> (w2653:string)
            n1164 = local read "S 39"() -> (w2664:string)
            n1165 = local read "String 34"() -> (w2666:string)
            n1166 = Concatenate Strings("6)" ("string"), w2656) -> (w2655:string)
            n1167 = Concatenate Strings("5)" ("string"), w2659) -> (w2658:string)
            n1168 = Concatenate Strings("4)" ("string"), w2661) -> (w2662:string)
            n1169 = Concatenate Strings("3)" ("string"), w2664) -> (w2665:string)
            n1170 = local read "S 38"() -> (w2671:string)
            n1171 = Concatenate Strings("2)" ("string"), w2666) -> (w2667:string)
            n1172 = Number To Fractional String(number=w2688, width (-)=i16 6, precision (6)=i16 2) -> (F-format string=w2687:string)  [unwired: 1 in]
            n1173 = Number To Fractional String(number=w2706, width (-)=i16 6, precision (6)=i16 2) -> (F-format string=w2708:string)  [unwired: 1 in]
            n1174 = Number To Fractional String(number=w2705, width (-)=i16 6, precision (6)=i16 2) -> (F-format string=w2707:string)  [unwired: 1 in]
            n1175 = Number To Fractional String(number=w2692, width (-)=i16 6, precision (6)=i16 2) -> (F-format string=w2693:string)  [unwired: 1 in]
            n1176 = Number To Fractional String(number=w2701, width (-)=i16 6, precision (6)=i16 2) -> (F-format string=w2704:string)  [unwired: 1 in]
            n1177 = Number To Fractional String(number=w2702, width (-)=i16 6, precision (6)=i16 2) -> (F-format string=w2691:string)  [unwired: 1 in]
            n1178 = Number To Fractional String(number=w2717, width (-)=i16 6, precision (6)=i16 2) -> (F-format string=w2722:string)  [unwired: 1 in]
            n1179 = call-poly <vilib>:"Append Report Text.vi"("report in"=w2700, "error in (no error)"=w2699) -> ("report out"=w2721:refnum<class "NI_report.lvclass">, "error out"=w2719:errorcluster)  [unwired: 10 in, 2 out]
            n1180 = local read "String 39"() -> (w2649:string)
            n1181 = local read "WS1.4 2"() -> (w2684:dbl)
            n1182 = Concatenate Strings("1)" ("string"), w2671) -> (w2670:string)
            n1183 = Concatenate Strings("8)" ("string"), w2649) -> (w2650:string)
            n1184 = Number To Fractional String(number=w2684, precision (6)=i16 2) -> (F-format string=w2683:string)  [unwired: 2 in]
            n1185 = Concatenate Strings(w2686, w2670, w2722, w2686, w2667, w2691, w2686, w2665, w2704, w2686, w2662, w2693, w2686, w2658, w2708, w2686, w2655, w2707, w2686, w2653, w2687, w2686, w2650, w2683) -> (w2674:string)
            "export 2" <- w2674
            n1186 = call-poly <vilib>:"Append Report Text.vi"("report in"=w2721, "text"=w2674, "error in (no error)"=w2719) -> ("report out"=w2720:refnum<class "NI_report.lvclass">, "error out"=w2718:errorcluster)  [unwired: 9 in, 2 out]
            n1187 = call-dynamic "Print Report.vi"("report in"=w2720, "printer name (default)"=w2728, "error in (no error)"=w2718) -> ("report out"=w2730:refnum<class "NI_report.lvclass">, "error out"=w2731:errorcluster)  [unwired: 11 in]
            n1188 = local read "test by"() -> (w2673:string)
            n1189 = local read "TITTLE"() -> (w2675:string)
            n1190 = local write "Print"(FALSE ("Print FF")) -> ()
            n1191 = call-dynamic "Dispose Report.vi"("report in"=w2730, "error in (no error)"=w2731) -> ()  [unwired: 13 in, 1 out]
            n1192 = Concatenate Strings(w2675, w2674, w2673) -> (→"output":string)
          }
        }
        n1193 = case shown="True" w2430 {
          frame False {
          }
          frame True {
            n1194 = flat-sequence {
              frame #0 {
              }
              frame #1 {
                n1195 = Wait (ms)(milliseconds to wait=u32 100) -> ()  [unwired: 1 out]
              }
              frame #2 {
